vi "heinzingerControlMain.vi"   [LabVIEW 2014]
uses:
  Controls/heinzingerSelect.ctl
  <vilib>/rvi/Emulation/niFpgaGetClockAttributes.vi
  <vilib>/rvi/Emulation/niFpgaSctlEmulationGetInTimedLoop.vi
  <vilib>/rvi/Emulation/niFpgaEmulationReportErrorSimple.vi
  <vilib>/rvi/eio/common/nirviEmuTemplateMethod_errors.vi
  <vilib>/rvi/Emulation/niFpgaCriticalErrorInLSC.vi
  <vilib>/eio/EIONode/EIONode.xnode
types:
  T1 = typedef "heinzingerSelect.ctl" = enum8{"Kepco", "Heinzinger0", "Heinzinger1", "Heinzinger2", "loading"}
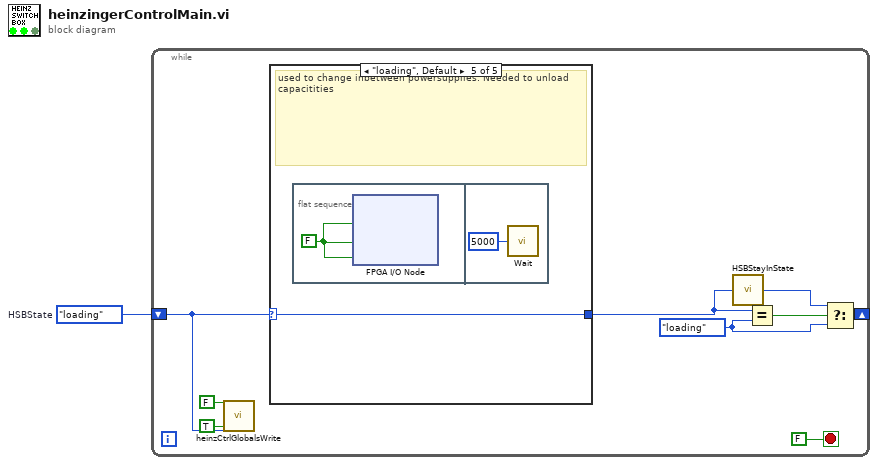
[diagram p0: block diagram]
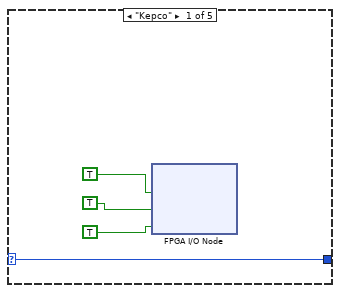
[diagram p2: hidden frame]
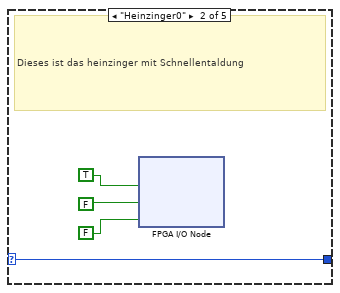
[diagram p3: hidden frame]
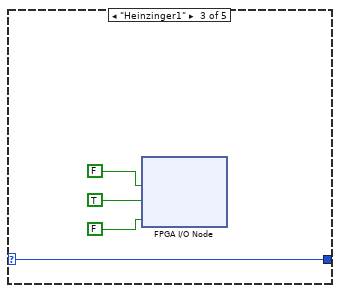
[diagram p4: hidden frame]
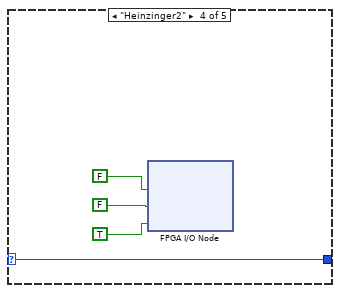
[diagram p5: hidden frame]
diagram:
  w1 = heinzingerSelect."loading"  # HSBState
  n1 = while {
    shift-right: [w6] -> _
    shift-left: w1 -> [w4]
    stop <- FALSE stop-if-true
    w8 = heinzingerSelect."loading" ("nextState")
    n2 = call "heinzCtrlGlobalsWrite.vi"("w_postAccOffsetVoltControl"=FALSE, "w_postAccOffsetVoltState"=TRUE, "postAccOffsetVoltState"=w4) -> ()  [unwired: 25 in]
    n3 = case shown="\"loading\", Default" w4 {
      selector: w4 -> [w14 w18 w22 w26 w27]
      tunnel: [w14 w18 w22 w26 w27] -> w5
      frame "Kepco" {
        n4 = xnode "FPGA I/O Node"("HeinzS0"=TRUE, "HeinzS1"=TRUE ("HeinzS0"), "HeinzS2"=TRUE ("HeinzS0")) -> ()  [unwired: 3 in, 3 out]
      }
      frame "Heinzinger0" {
        # "Dieses ist das heinzinger mit Schnellentaldung"
        n5 = xnode "FPGA I/O Node"("HeinzS0"=TRUE, "HeinzS1"=FALSE ("HeinzS0"), "HeinzS2"=FALSE ("HeinzS0")) -> ()  [unwired: 3 in, 3 out]
      }
      frame "Heinzinger1" {
        n6 = xnode "FPGA I/O Node"("HeinzS0"=FALSE, "HeinzS1"=TRUE ("HeinzS0"), "HeinzS2"=FALSE ("HeinzS0")) -> ()  [unwired: 3 in, 3 out]
      }
      frame "Heinzinger2" {
        n7 = xnode "FPGA I/O Node"("HeinzS0"=FALSE, "HeinzS1"=FALSE ("HeinzS0"), "HeinzS2"=TRUE ("HeinzS0")) -> ()  [unwired: 3 in, 3 out]
      }
      frame "loading", Default {
        # "used to change inbetween powersupplies. Needed to unload capacitities"
        n8 = flat-sequence {
          frame #0 {
            w28 = FALSE ("HeinzS0")
            n9 = xnode "FPGA I/O Node"("HeinzS0"=w28, "HeinzS1"=w28, "HeinzS2"=w28) -> ()  [unwired: 3 in, 3 out]
          }
          frame #1 {
            n10 = call "Wait"("Count(mSec)"=u32 5000) -> ()  [unwired: 1 out]
          }
        }
      }
    }
    n11 = call "HSBStayInState.vi"("lastCmd"=w5) -> ("newHSBCmd"=w7:T1)  [unwired: 14 in]
    n12 = Equal?(x=w5, y=w8) -> (x = y?=w9:bool)
    n13 = Select(t=w7, s=w9, f=w8) -> (s? t:f=w6:T1)
  }
